vi "TDMS Upload Example (Time Channel).vi"() -> ()   [LabVIEW 2024]
doc: "TDMS upload example."
uses:
  Sift API/Sift Client.lvclass
  Sift API/Types/TDMS Time Format.ctl
  Sift Client.lvlib
panel:
  in  "API gRPC URL":string
  in  "Run Name":string="TDMS Upload Example"
  in  "Asset Name":string="LabVIEW-TDMS-Example"
  in  "Absolute Filepath":path
  out "Error":errorcluster
  in  "API Key":string
  in  "API REST URL":string
  # "Instructions\n\n1. Fill in the API URLs and API Key. Visit this URL for more information on authentication\n    https://docs.siftstack.com/docs/api/authentication\n\n2. Select a TDMS file to upload. There is a \"sample_data.tdms\" file in the same Example directory of this VI.\n\n3. Run the VI.\n\n3. The VI should run to completetion with no errors. Navigate to the Sift home page and find the \n     Run to see the example data."
  # "Sift TDMS Upload Example (Time Channel)"
  # "Run this example to test uploading TDMS files to Sift. This is for TDMS\nformats that contain a dedicated Time channel within each group."
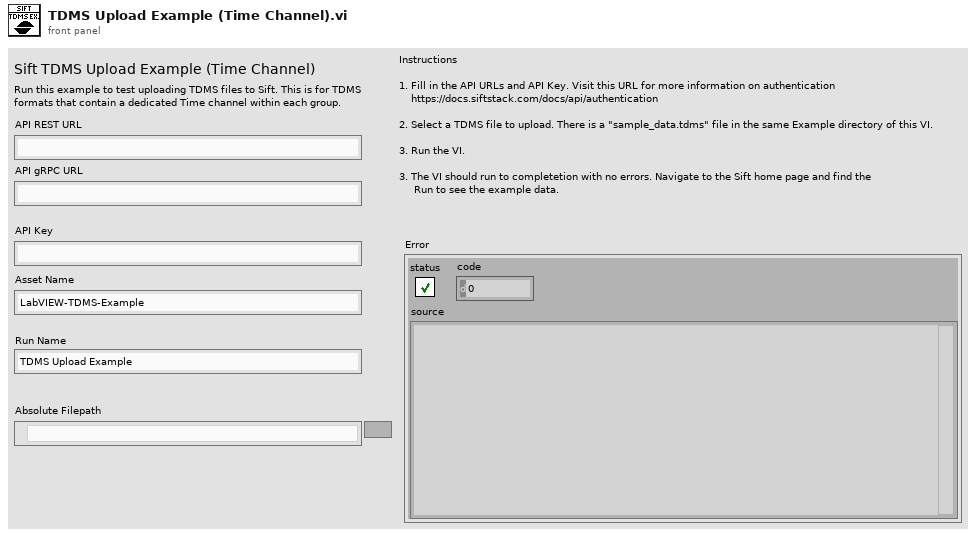
[diagram p1: front panel]
types:
  T1 = typedef "Sift Client.lvlib/TDMS Time Format.ctl" = enum16{"waveform", "time_channel"}
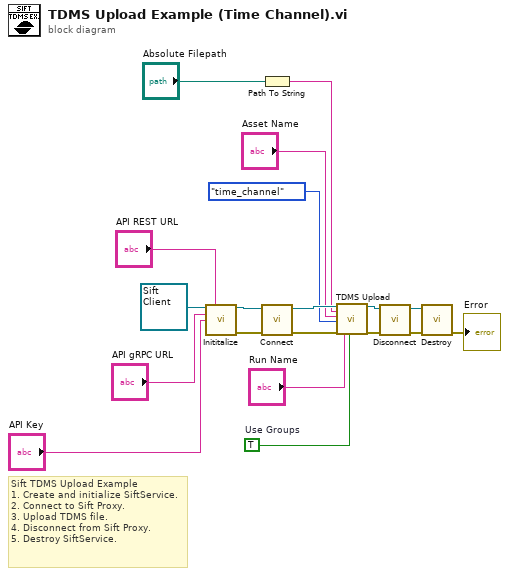
[diagram p0: block diagram]
diagram:
  w3 = TRUE  # Use Groups
  # "Sift TDMS Upload Example\n1. Create and initialize SiftService.\n2. Connect to Sift Proxy.\n3. Upload TDMS file.\n4. Disconnect from Sift Proxy.\n5. Destroy SiftService."
  n1 = call-dynamic "Inititalize.vi"("Sift Client in"=refnum<class "Sift Client.lvclass"> refnum ("Sift Client.lvlib:Sift Client.lvclass"), "REST URL"="API REST URL", "GRPC URL"="API gRPC URL", "API Key"="API Key") -> ("Sift Client out"=w16:refnum<class "Sift Client.lvclass">, "error out"=w15:errorcluster)  [unwired: 10 in]
  n2 = Path To String(path="Absolute Filepath") -> (string=w6:string)
  n3 = call-dynamic "Connect.vi"("error in (no error)"=w15, "Sift Client in"=w16) -> ("error out"=w13:errorcluster, "Sift Client out"=w14:refnum<class "Sift Client.lvclass">)  [unwired: 7 in, 1 out]
  n4 = call-dynamic "TDMS Upload.vi"("Sift Client in"=w14, "Filepath"=w6, "Asset Name"="Asset Name", "TDMS Time Format"=TDMS_Time_Format."time_channel" ("Enum"), "error in (no error)"=w13, "Run Name"="Run Name", "Group Into Components"=w3) -> ("Sift Client out"=w12:refnum<class "Sift Client.lvclass">, "error out"=w11:errorcluster)  [unwired: 11 in]
  n5 = call-dynamic "Disconnect.vi"("error in (no error)"=w11, "Sift Client in"=w12) -> ("error out"=w9:errorcluster, "Sift Client out"=w10:refnum<class "Sift Client.lvclass">)  [unwired: 8 in]
  n6 = call-dynamic "Destroy.vi"("error in (no error)"=w9, "Sift Client in"=w10) -> ("error out"=→"Error":errorcluster)  [unwired: 8 in, 1 out]
